vi "Convert.I16toFXP.vi"(4 "16bit integer":i16) -> (1 "x*y":fxp<+/-,20,5>)   [LabVIEW 2015, in "FPGA Wizard Templates.lvlib"]
uses:
  FPGA Wizard Templates.lvlib
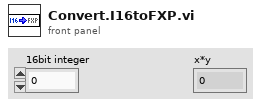
[diagram p1: front panel]
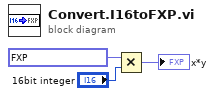
[diagram p0: block diagram]
diagram:
  n1 = Multiply(x=fxp<+/-,16,1> 0.00030517578125 ("Connector1/AO0"), y="16bit integer") -> (x*y=→"x*y":fxp<+/-,20,5>)
